vi "compare readings R140.vi"() -> ()   [LabVIEW 2020]
uses:
  common/record_file_handler/VFH-VNA_File_Handler.lvlib
panel:
  out "appended path":path
  out "All Files in Dir":path[](array[path])
  in  "Tab Control":enum32{"Page 1", "Page 3", "Page 2"}(tab)
  in  "Max range":dbl
  in  "min range":dbl
  out "Ref R":cluster{"Frequency":dbl[], "S21_Imag":dbl[]}[](graph)
  out "Ref I":cluster{"Frequency":dbl[], "S21_Imag":dbl[]}[](graph)
  out "p'":cluster{"Frequency":dbl[], "S21_Imag":dbl[]}[](graph)
  out "p''":cluster{"Frequency":dbl[], "S21_Imag":dbl[]}[](graph)
  in  "Stop":bool
  in  "Max range 2":dbl
  in  "min range 2":dbl
  out "Tan":cluster{"Frequency":dbl[], "S21_Imag":dbl[]}[](graph)
  out "Q [S/m]":cluster{"Frequency":dbl[], "S21_Imag":dbl[]}[](graph)
  in  "Stop 2":bool
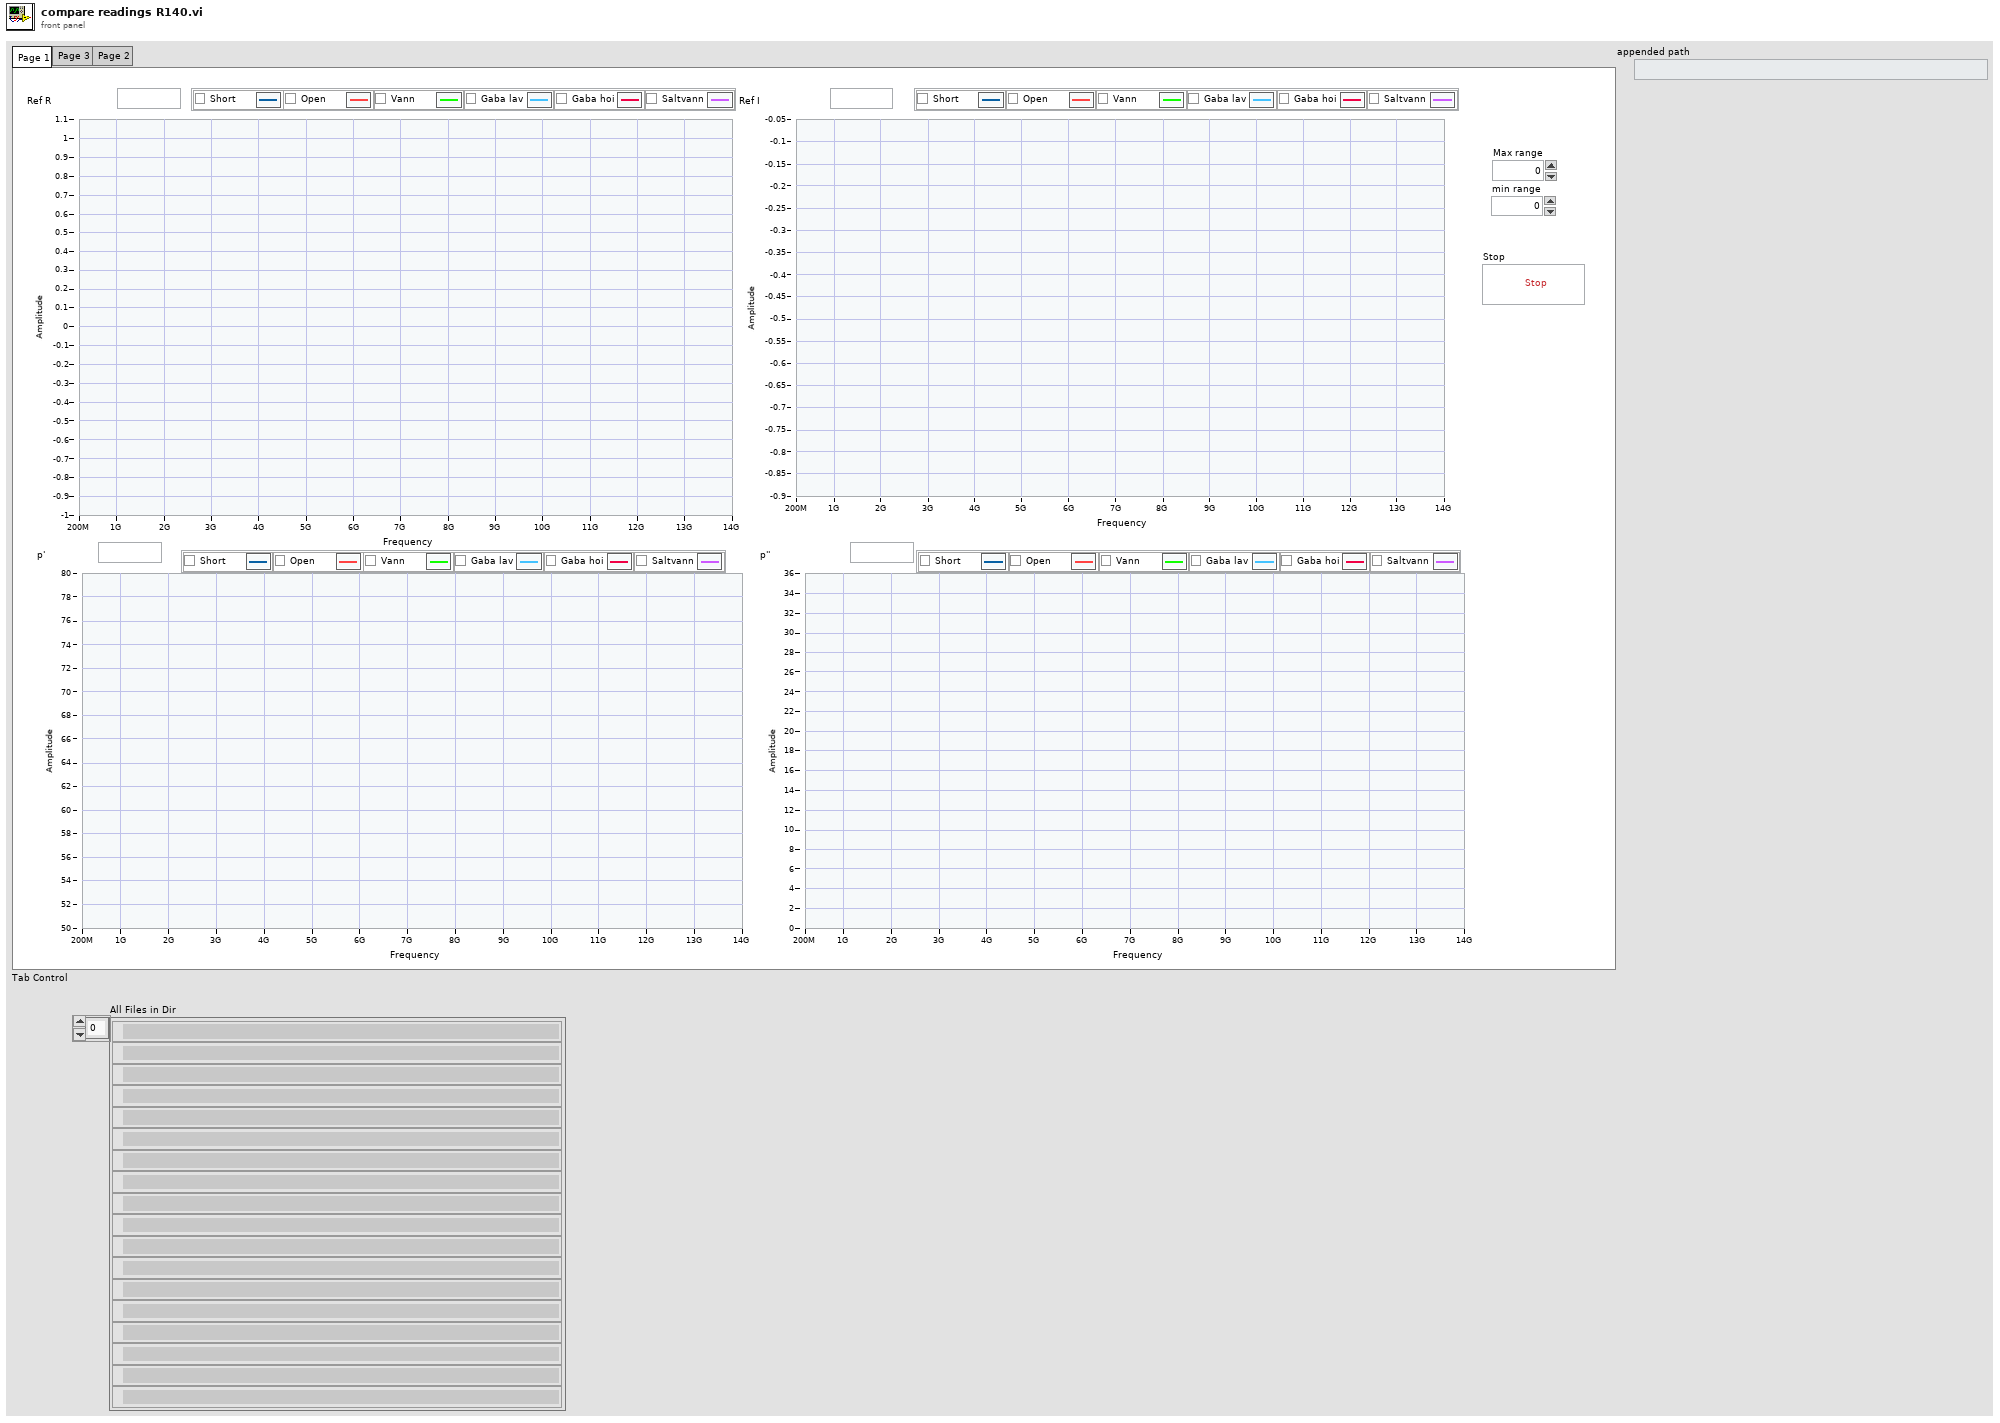
[diagram p1: front panel]
types:
  T1 = typedef "VFH-VNA_File_Handler.lvlib/VFH-file_cluster-Expensive.ctl" = cluster{"Frequency":dbl[], "Permativity'":dbl[], "Permativity''":dbl[], "Q [S/m]":dbl[], "Tan":dbl[], "Reflection R":dbl[], "Reflection I":dbl[]}
  T2 = cluster{"Frequency":dbl[], "Permativity''":dbl[]}
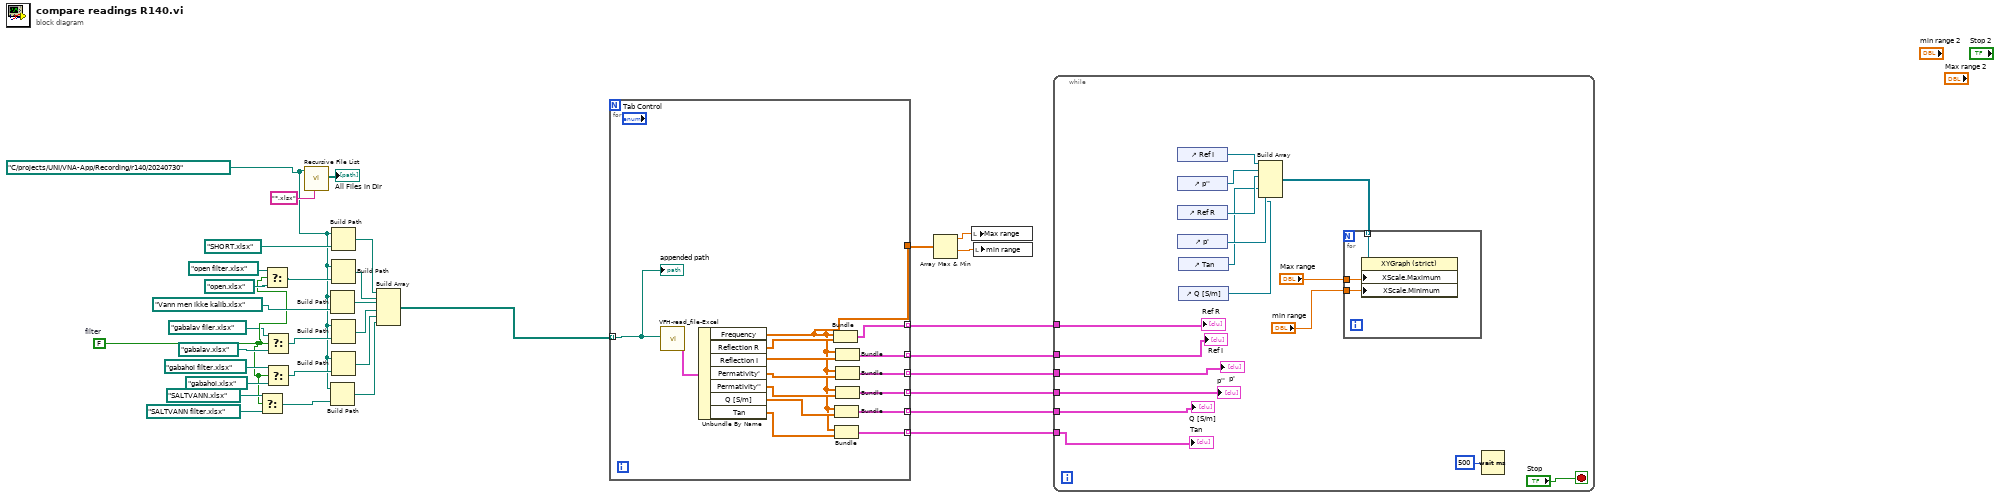
[diagram p0: block diagram]
diagram:
  w6 = FALSE  # filter
  w1 = path "C:/projects/UNI/VNA-App/Recording/r140/20240730" ("Folder Path")
  n1 = Select(t=path "SALTVANN.xlsx" ("name or relative path"), s=w6, f=path "SALTVANN filter.xlsx" ("name or relative path")) -> (s? t:f=w10:path)
  n2 = Select(t=path "open filter.xlsx" ("name or relative path"), s=w6, f=path "open.xlsx" ("name or relative path")) -> (s? t:f=w8:path)
  n3 = Select(t=path "gabalav filer.xlsx" ("name or relative path"), s=w6, f=path "gabalav.xlsx" ("name or relative path")) -> (s? t:f=w5:path)
  n4 = Select(t=path "gabahoi filter.xlsx" ("name or relative path"), s=w6, f=path "gabahoi.xlsx" ("name or relative path")) -> (s? t:f=w13:path)
  n5 = call <vilib>:"Recursive File List.vi"("pattern"="*.xlsx", "Folder Path"=w1) -> ("All Files in Dir"=→"All Files in Dir":path[])  [unwired: 5 in, 4 out]
  n6 = Build Path(base path=w1, name or relative path=path "Vann men ikke kalib.xlsx") -> (appended path=w23:path)
  n7 = Build Path(base path=w1, name or relative path=w10) -> (appended path=w20:path)
  n8 = Build Path(base path=w1, name or relative path=path "SHORT.xlsx") -> (appended path=w25:path)
  n9 = Build Path(base path=w1, name or relative path=w8) -> (appended path=w24:path)
  n10 = Build Path(base path=w1, name or relative path=w5) -> (appended path=w22:path)
  n11 = Build Path(base path=w1, name or relative path=w13) -> (appended path=w21:path)
  n12 = Build Array(w25, w24, w23, w22, w21, w20) -> (w18:path[])
  n13 = for {
    tunnel: w18 -> [w49] mode=indexing
    tunnel: [w43] -> w34 mode=indexing
    tunnel: [w42] -> w33 mode=indexing
    tunnel: [w41] -> w32 mode=indexing
    tunnel: [w40] -> w31 mode=indexing
    tunnel: [w37] -> w30
    tunnel: [w36] -> w27 mode=indexing
    tunnel: [w35] -> w26 mode=indexing
    n14 = call "VFH-read_file-Excel.vi"("file path (dialog if empty)"=w49) -> ("output cluster"=w48:T1)  [unwired: 9 in, 1 out]
    n15 = Unbundle By Name(w48) -> ("Frequency"=w37:dbl[], "Reflection R"=w47:dbl[], "Reflection I"=w46:dbl[], "Permativity'"=w45:dbl[], "Permativity''"=w44:dbl[], "Q [S/m]"=w38:dbl[], "Tan"=w39:dbl[])
    n16 = Bundle("Frequency"=w37, "Reflection R"=w47) -> (w43:cluster{"Frequency":dbl[], "Reflection R":dbl[]})  [unwired: 1 in]
    n17 = Bundle("Frequency"=w37, "Tan"=w39) -> (w35:cluster{"Frequency":dbl[], "Tan":dbl[]})  [unwired: 1 in]
    n18 = Bundle("Frequency"=w37, "Q [S/m]"=w38) -> (w36:cluster{"Frequency":dbl[], "Q [S/m]":dbl[]})  [unwired: 1 in]
    n19 = Bundle("Frequency"=w37, "Reflection I"=w46) -> (w42:cluster{"Frequency":dbl[], "Reflection I":dbl[]})  [unwired: 1 in]
    n20 = Bundle("Frequency"=w37, "Permativity'"=w45) -> (w41:cluster{"Frequency":dbl[], "Permativity'":dbl[]})  [unwired: 1 in]
    n21 = Bundle("Frequency"=w37, "Permativity''"=w44) -> (w40:T2)  [unwired: 1 in]
    "appended path" <- w49
  }
  n22 = Array Max & Min(array=w30) -> (max value=w29:dbl, min value=w28:dbl)  [unwired: 2 out]
  n23 = local write "Max range"(w29) -> ()
  n24 = local write "min range"(w28) -> ()
  n25 = while {
    tunnel: w34 -> [w64]
    tunnel: w33 -> [w63]
    tunnel: w32 -> [w62]
    tunnel: w31 -> [w61]
    tunnel: w27 -> [w53]
    tunnel: w26 -> [w52]
    stop <- "Stop" stop-if-true
    n26 = control-ref of="Ref I"() -> (w60:refnum<vi>)
    n27 = control-ref of="p''"() -> (w59:refnum<vi>)
    n28 = control-ref of="Ref R"() -> (w58:refnum<vi>)
    n29 = control-ref of="p'"() -> (w57:refnum<vi>)
    n30 = control-ref of="Tan"() -> (w51:refnum<vi>)
    n31 = control-ref of="Q [S/m]"() -> (w50:refnum<vi>)
    n32 = Build Array(w60, w59, w58, w57, w51, w50) -> (w56:refnum<vi>[])
    n33 = for {
      tunnel: w56 -> [w69] mode=indexing
      tunnel: "Max range" -> [w68]
      tunnel: "min range" -> [w67]
      n34 = property class="XYGraph (strict)"(reference=w69, "XScale.Maximum"=w68, "XScale.Minimum"=w67) -> ()  [unwired: 1 in, 2 out]
    }
    n35 = Wait (ms)(milliseconds to wait=u32 500) -> ()  [unwired: 1 out]
    "p'" <- w62
    "Ref R" <- w64
    "p''" <- w61
    "Ref I" <- w63
    "Q [S/m]" <- w53
    "Tan" <- w52
  }
